vi "Read_DriveCommand.vi"(8 "error in (no error)":errorcluster, 11 "DriveData in":refnum<class "DriveData.lvclass">) -> (0 "error out":errorcluster, 2 "DriveCommand":T1, 3 "DriveData out":refnum<class "DriveData.lvclass">)   [LabVIEW 2017, in "DriveData.lvclass"]
uses:
  DriveData.lvclass
  DriveCommand.ctl
  DriveData.lvclass/DriveData.ctl
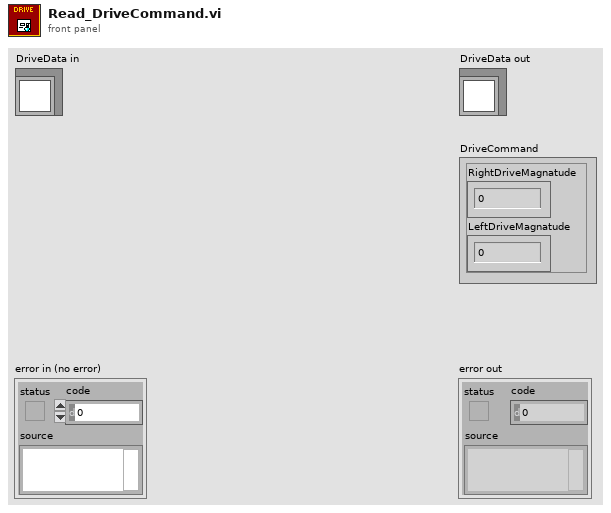
[diagram p1: front panel]
types:
  T1 = typedef "DriveData.lvclass/DriveCommand.ctl" = cluster{"RightDriveMagnatude":dbl, "LeftDriveMagnatude":dbl}
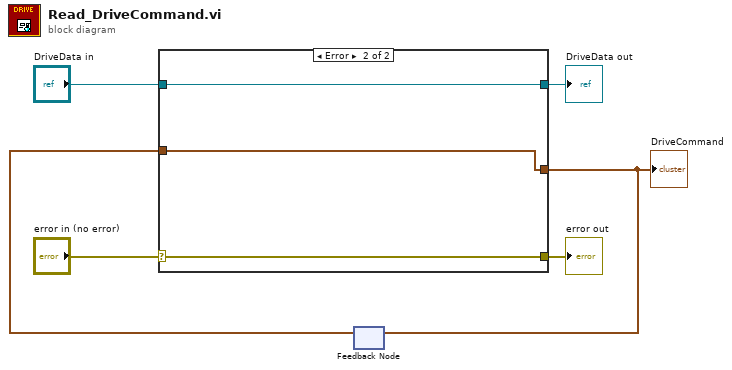
[diagram p0: block diagram]
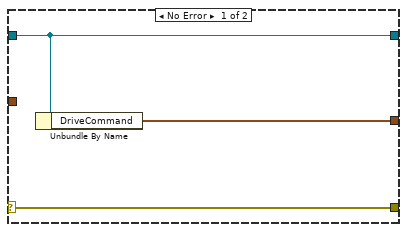
[diagram p2: hidden frame]
diagram:
  n1 = feedback #1() -> (w1:T1)  [unwired: 1 in]
  n2 = case shown="Error" "error in (no error)" {
    selector: "error in (no error)" -> [w9 w11]
    tunnel: [w9 w11] -> w5
    tunnel: [w8 w12] -> w3
    tunnel: "DriveData in" -> [w8 w12]
    tunnel: [w7 w10] -> w2
    tunnel: w1 -> [_ w10]
    frame No Error {
      n3 = Unbundle By Name(w8) -> ("DriveCommand"=w7:T1)
    }
    frame Error {
    }
  }
  "error out" <- w5
  "DriveData out" <- w3
  "DriveCommand" <- w2
  n4 = feedback-in #1(w2) -> ()
